vi "Add Tip Offset.vi"(11 "XYZTheta":dbl[](array[numeric])) -> (3 "XYZTheta":dbl[](array[numeric]))   [LabVIEW 2021, in "Dispense.lvclass"]
uses:
  Dispense.lvclass
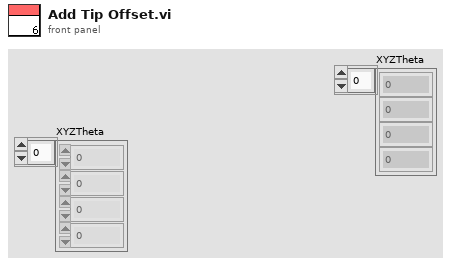
[diagram p1: front panel]
types:
  T1 = typedef "File Paths.ctl" = cluster{"Glue Pattern Folder":path, "Carrier Tray Folder":path, "Pick Up Tool Fixture Folder":path, "Components Folder":path, "Bellows Tool Offset.txt":path, "Pick Up Tool Offset.txt":path, "Dispense Tip Offset.txt":path, "Log Files":path, "Gantry Assembly Map.txt":path, "Syringe and offset map.txt":path, "Controllers Folder":path, "Local dbase config":path}
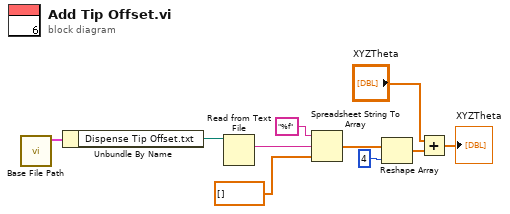
[diagram p0: block diagram]
diagram:
  n1 = call "Base File Path.vi"() -> ("Paths Out"=w9:T1)  [unwired: 11 in]
  n2 = Unbundle By Name(w9) -> ("Dispense Tip Offset.txt"=w10:path)
  n3 = Read from Text File(file (use dialog)=w10) -> (text=w7:string)  [unwired: 3 in, 3 out]
  n4 = Spreadsheet String To Array(format string="%f", spreadsheet string=w7, array type (2D Dbl)=dbl[] []) -> (array=w3:dbl[])  [unwired: 1 in]
  n5 = Reshape Array(w3, 4 ("dimension size")) -> (w4:dbl[])
  n6 = Add(x="XYZTheta", y=w4) -> (x+y=→"XYZTheta":dbl[])
